vi "SA40144D.20210601 Devices + BG.vi"() -> ()   [LabVIEW 2020]
uses:
  <vilib>/Analysis/baseanly.llb/Mean (DBL).vi
  <userlib>/_OpenG.lib/file/file.llb/Build Path - Traditional__ogtk.vi
  <userlib>/LevyLab/LV to ITX/Data/Data.lvclass
  <userlib>/LevyLab/XY Utilities/xy_utilities.lvlib
  <vilib>/Analysis/NI_AALBase.lvlib
panel:
  in  "Tab Control":enum32{"Page 1", "Page 2", "Page 3"}(tab)
  out "G2T BG vs t":T1(graph)
  out "Temp vs t":T1(graph)
  out "G2T vs t 1D":T1(graph)
  out "G4T vs t 1D":T1(graph)
  out "G2T vs t 2D":T1(graph)
  out "G4T vs t  2D":T1(graph)
  out "Arrhenius":T1(graph)
  out "Lifespan vs Temp (hrs)":cluster{i32[], dbl[]}[](graph)
  out "Y3 2D I-":T1(graph)
  out "Y1 - BG I+":T1(graph)
  out "Y2 - 2D I+":T1(graph)
  out "Y4 - 1D I+":T1(graph)
  out "R3 - 2D I-":T1(graph)
  out "X3 - 2D I-":T1(graph)
  out "X2 - 2D I+":T1(graph)
  out "R1 - BG I+":T1(graph)
  out "X1 - BG I+":T1(graph)
  out "X4 - 1D I+":T1(graph)
  out "R2 - 2D I+":T1(graph)
  out "R4 - 1D I+":T1(graph)
  out "Y6 - 2D dV":T1(graph)
  out "Y8 - BG I-":T1(graph)
  out "Y5 - 1D I-":T1(graph)
  out "Y7 - 1D dV":T1(graph)
  out "R6 - 2D dV":T1(graph)
  out "R8 - BG I-":T1(graph)
  out "X5 - 1D I-":T1(graph)
  out "R5 - 1D I-":T1(graph)
  out "X6 - 2D dV":T1(graph)
  out "X7 - 1D dV":T1(graph)
  out "R7 - 1D dV":T1(graph)
  out "X8 - BG I-":T1(graph)
  in  "Toggle":bool
  in  "Temps to keep (Lifespan)":i32=26
  out "E_a":dbl[](array[numeric])
  in  "Temps to keep (Arrhenius fit)":i32=26
  in  "Source Voltage":dbl=0.1
  in  "Init Temp":i32=275
  in  "Temp Step":i32=5
  in  "Final Temp":i32=400
  in  "Data File":path=path "G:/My Drive/ansom/Data/PPMS 2/SA40144D.20210601/00 - Air Test/SA40144D.20210601.275K.dat"
  in  "Trimming":i32=400
  in  "Update":bool
  in  "OK":bool
  out "error out":errorcluster
  in  "error in (no error)":errorcluster
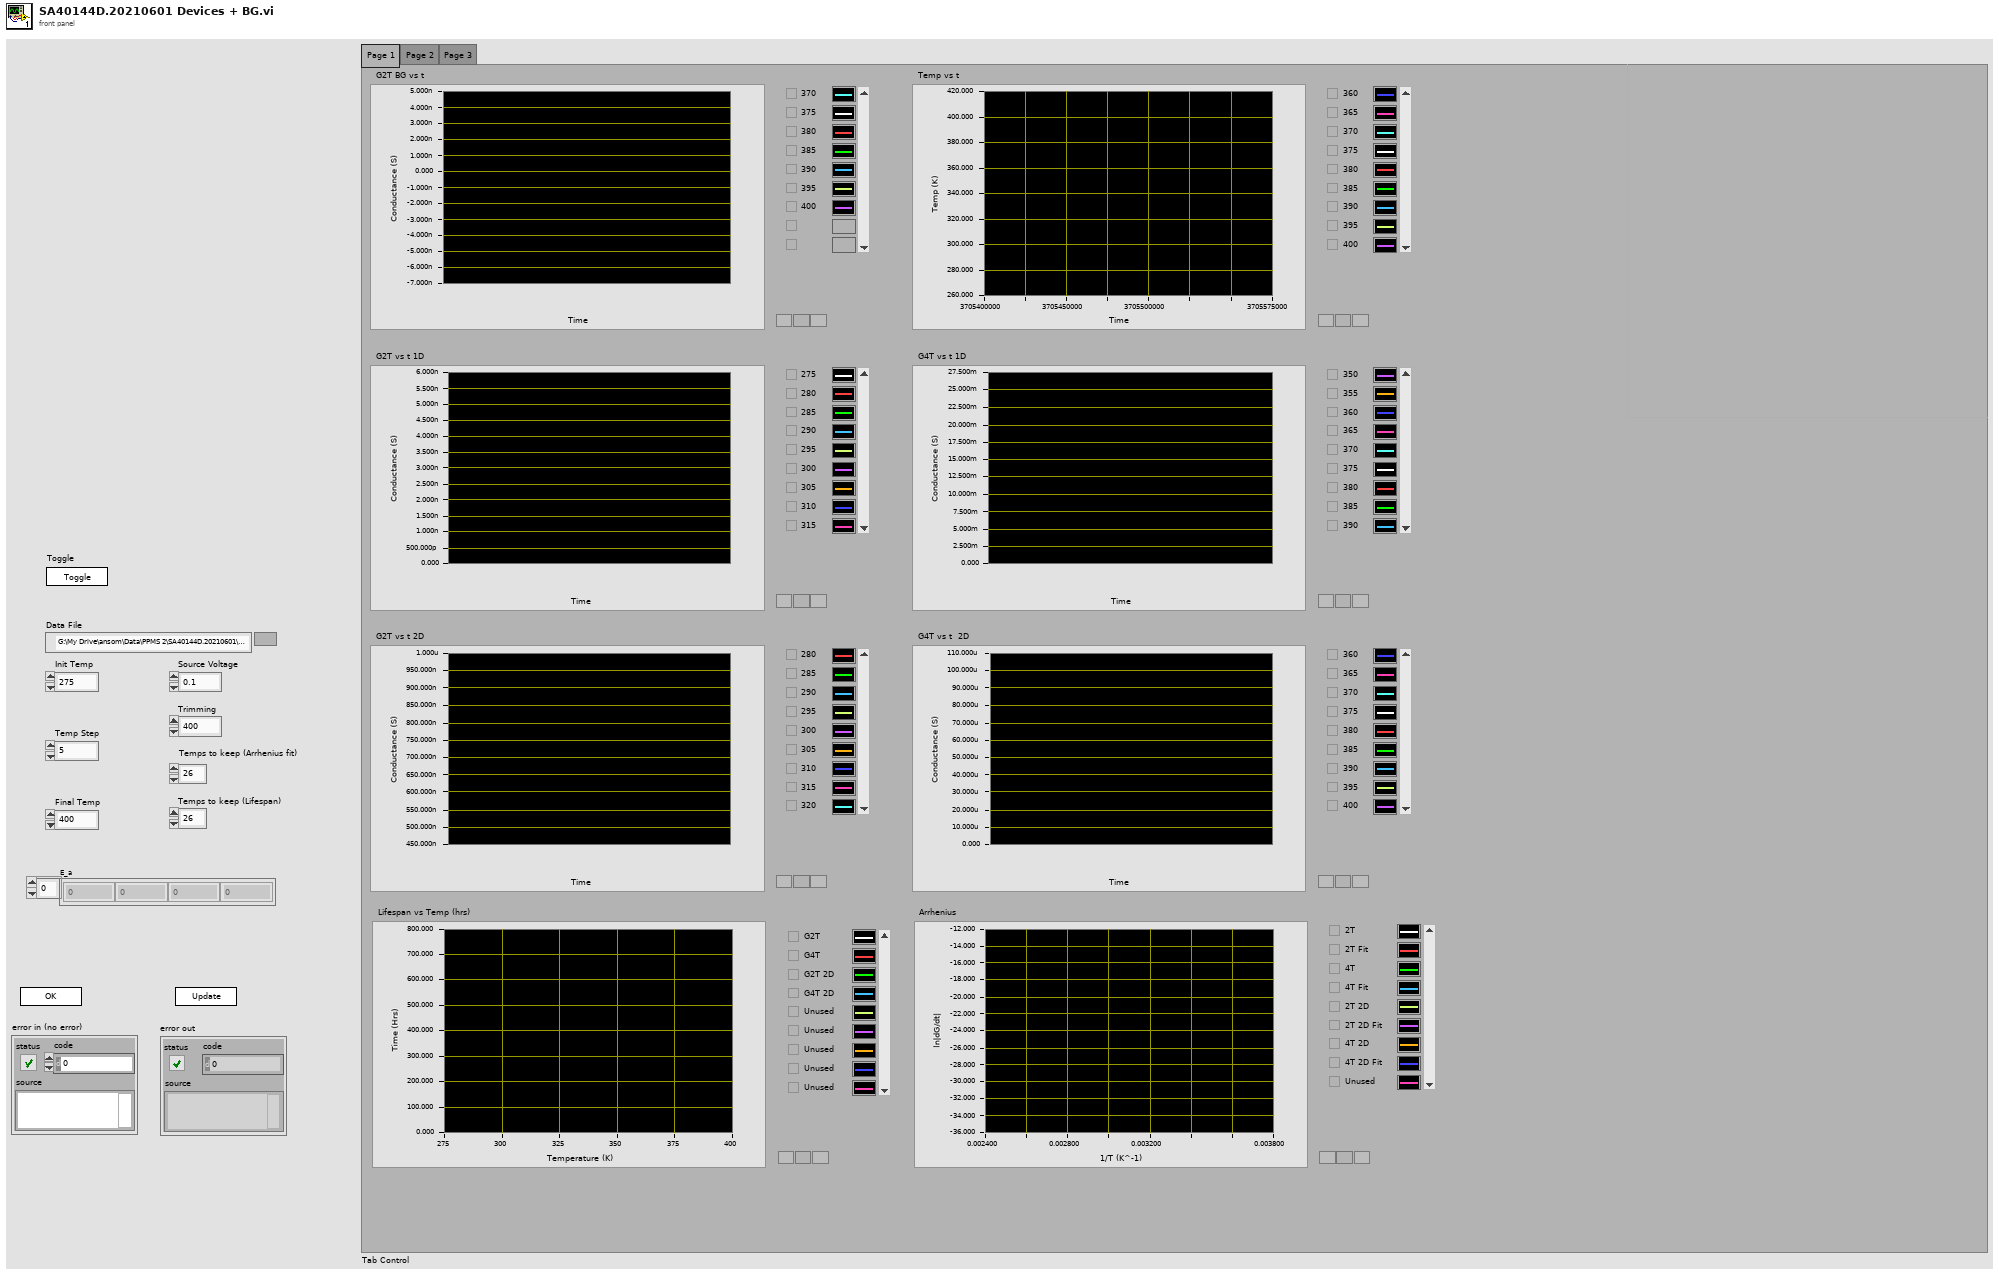
[diagram p1: front panel]
types:
  T1 = cluster{"Data":dbl[], "Best Exponential Fit":dbl[]}[]
  T2 = enum32{"Invalid", "Standard", "Closed", "Hidden", "Minimized", "Maximized"}
  T3 = enum32{"invalid app kind", "Development System", "Run Time System", "Student Edition", "Embedded LabVIEW", "Evaluation", "Custom"}
  T4 = cluster{"Core":cluster{"Current VI Reference":refnum<vi>, "Close Panel on Exit?":bool}, "G2T 1D":cluster{dbl[], dbl[]}[], "G4T 1D":cluster{dbl[], dbl[]}[], "G2T 2D":cluster{dbl[], dbl[]}[], "G4T 2D":cluster{dbl[], dbl[]}[], "Temp":cluster{dbl[], dbl[]}[], "G2T BG":cluster{dbl[], dbl[]}[], "Source Voltage":dbl, "Final Temp":i32, "Init Temp":i32, "Temp Step":i32, "Data File":path, "Trimming":i32}
  T5 = cluster{"Current VI Reference":refnum<vi>, "Close Panel on Exit?":bool}
  T6 = typedef "Data.lvclass/Dictionary--cluster.ctl" = cluster{"key":string, "value":variant}
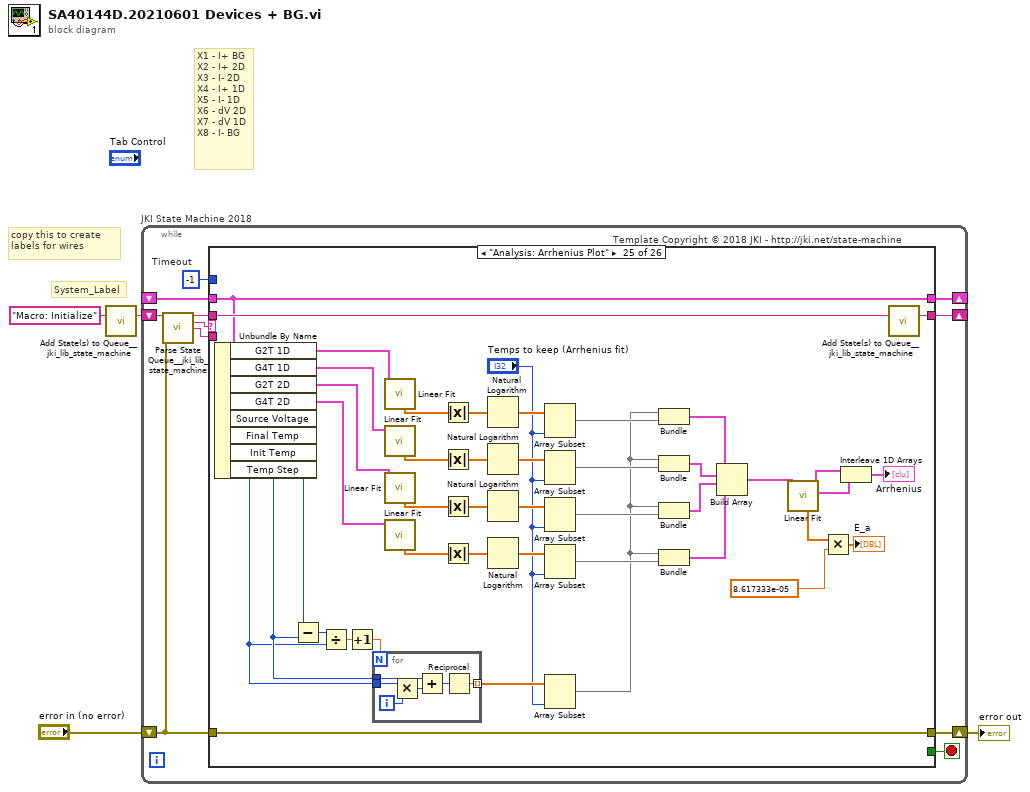
[diagram p0: block diagram]
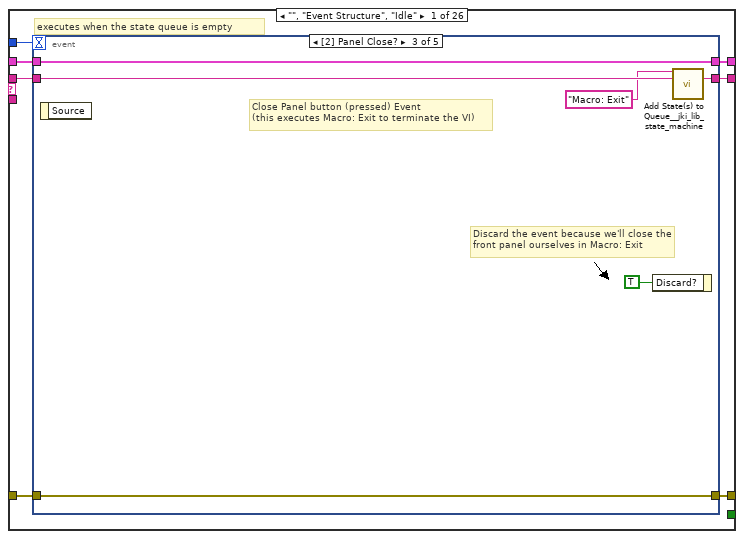
[diagram p2: hidden frame]
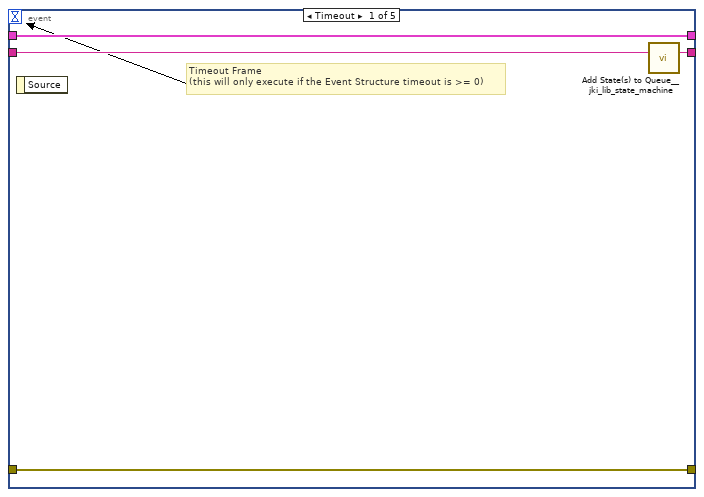
[diagram p3: hidden frame]
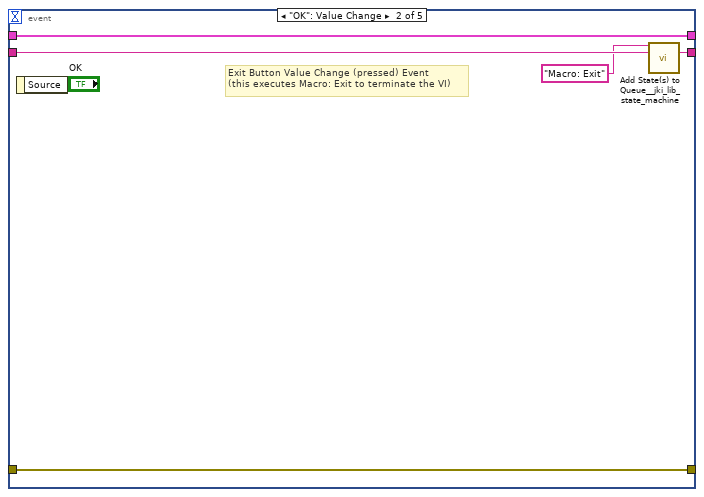
[diagram p4: hidden frame]
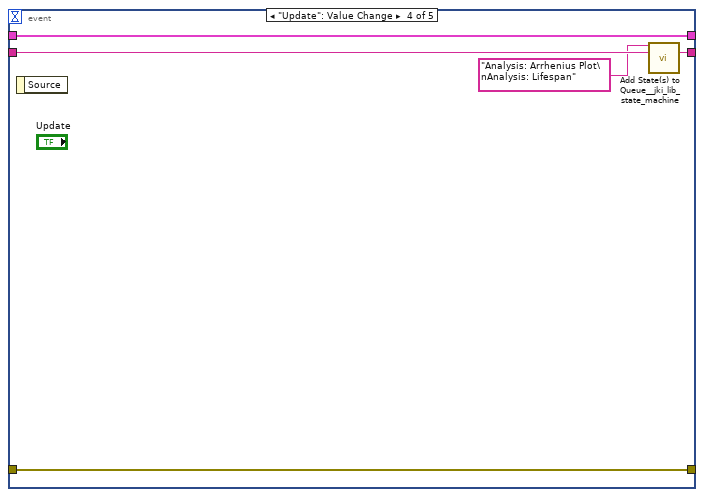
[diagram p5: hidden frame]
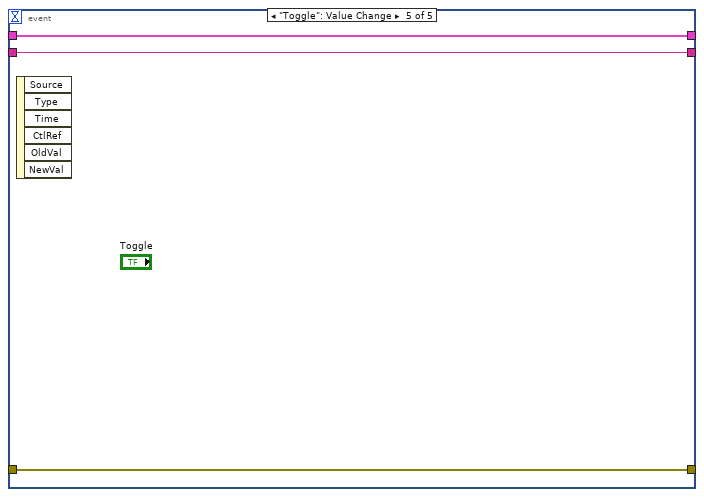
[diagram p6: hidden frame]
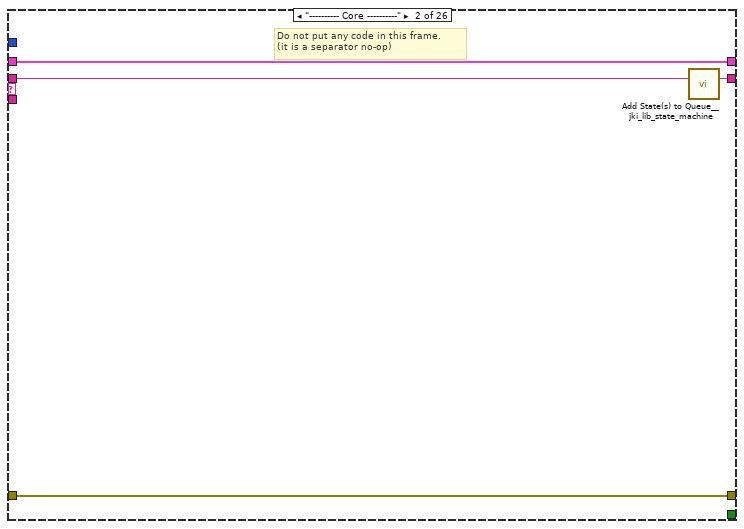
[diagram p7: hidden frame]
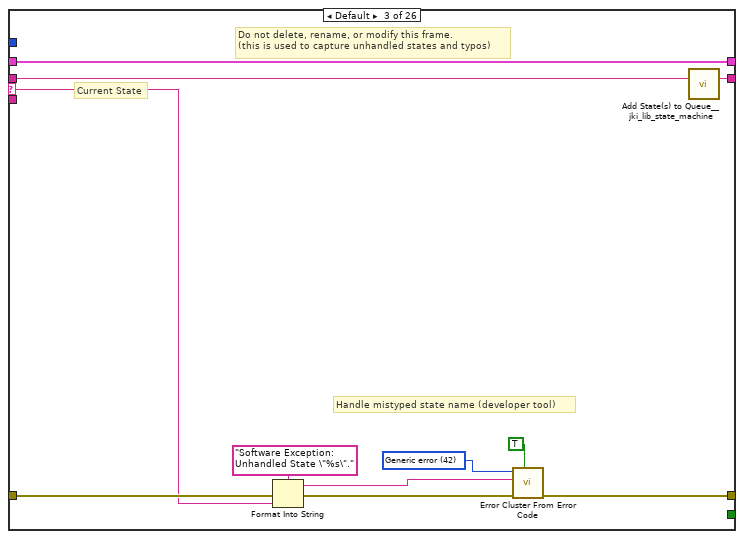
[diagram p8: hidden frame]
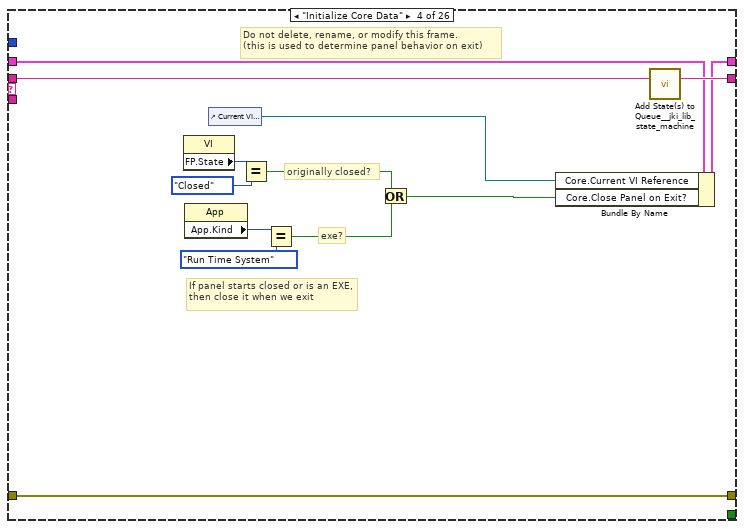
[diagram p9: hidden frame]
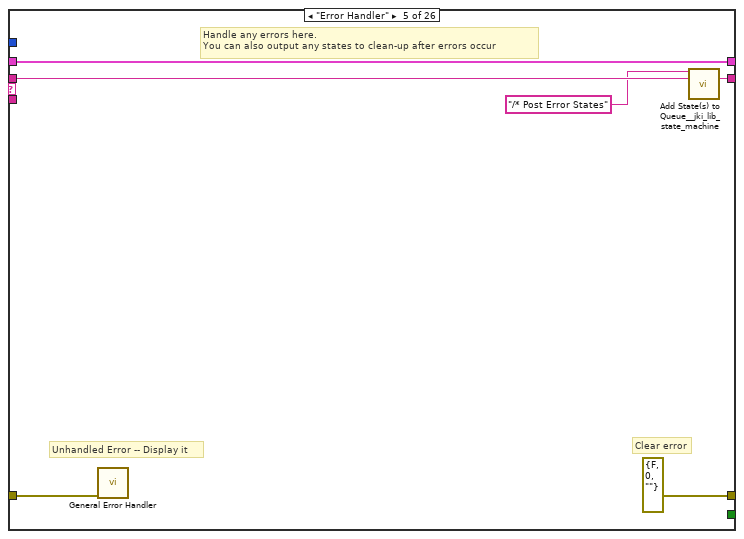
[diagram p10: hidden frame]
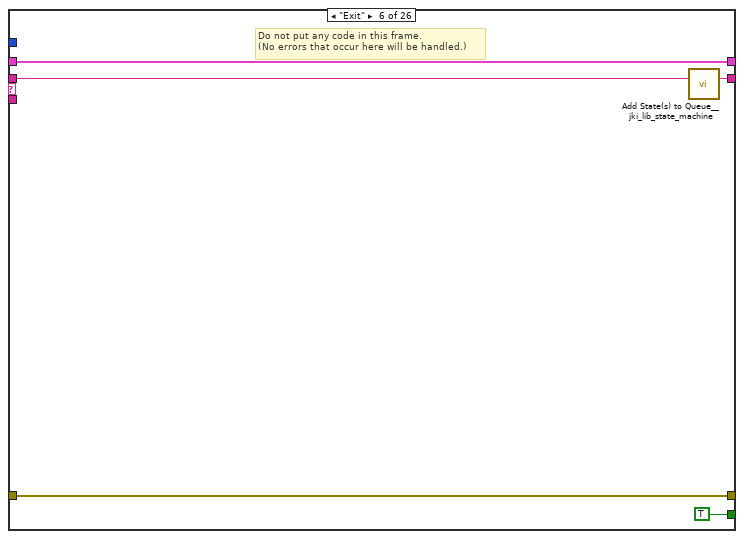
[diagram p11: hidden frame]
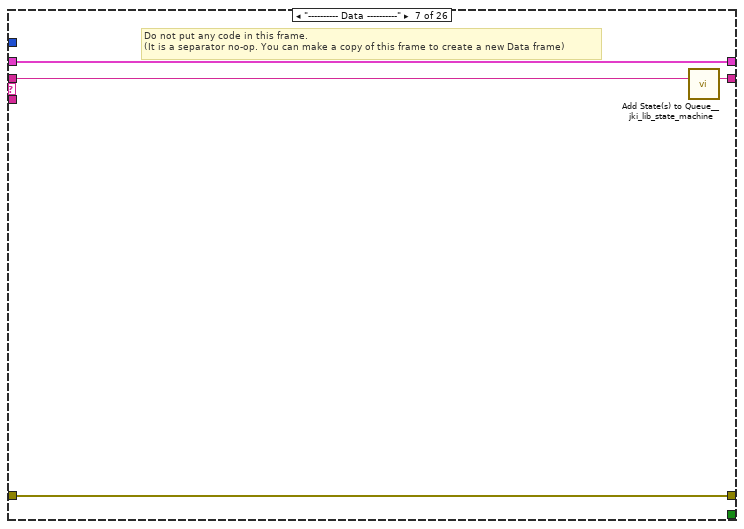
[diagram p12: hidden frame]
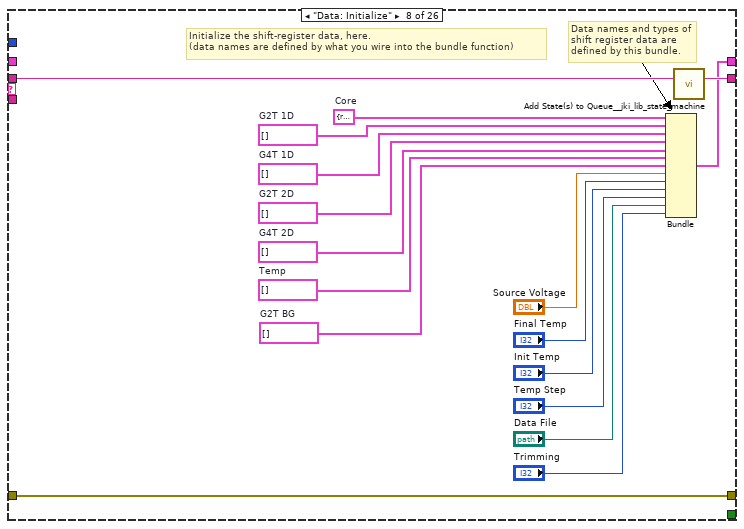
[diagram p13: hidden frame]
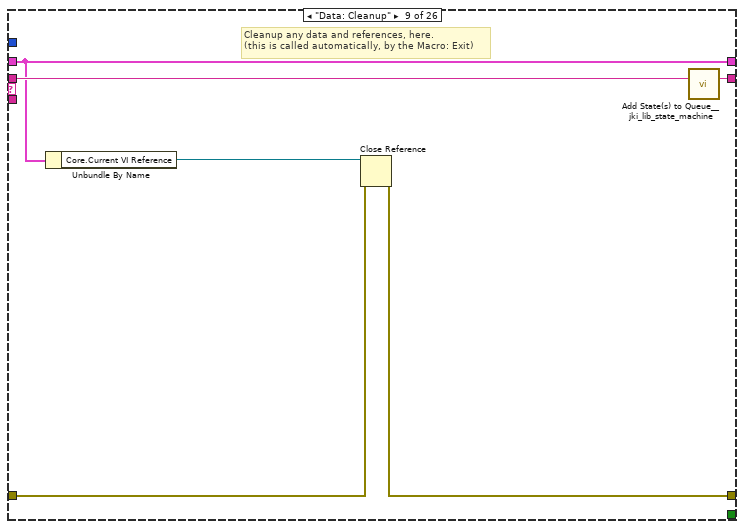
[diagram p14: hidden frame]
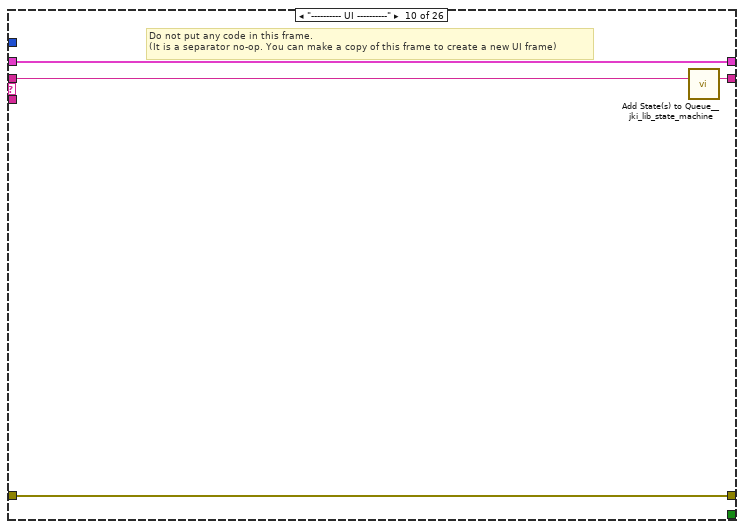
[diagram p15: hidden frame]
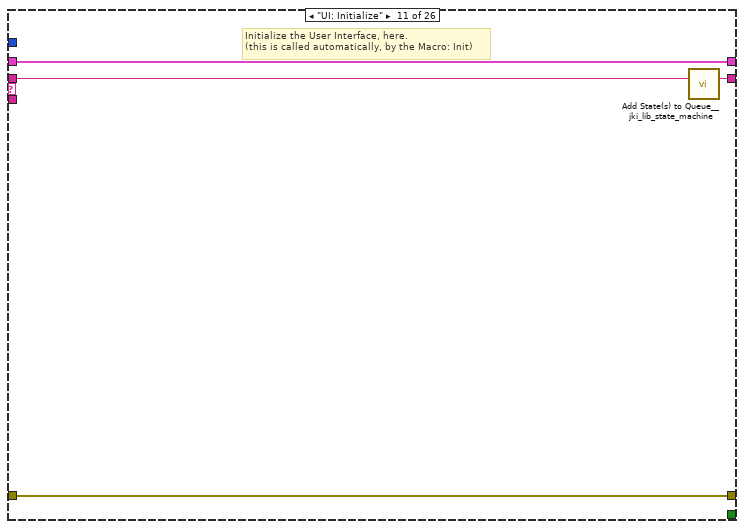
[diagram p16: hidden frame]
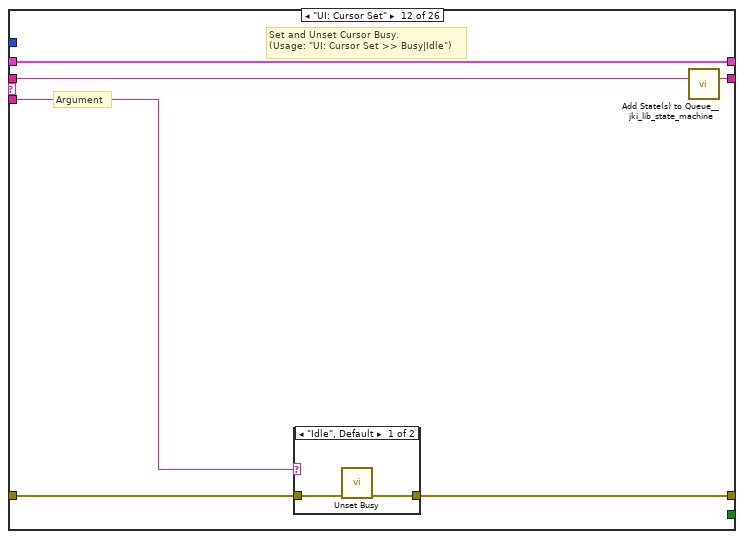
[diagram p17: hidden frame]
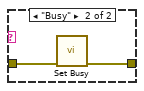
[diagram p18: hidden frame]
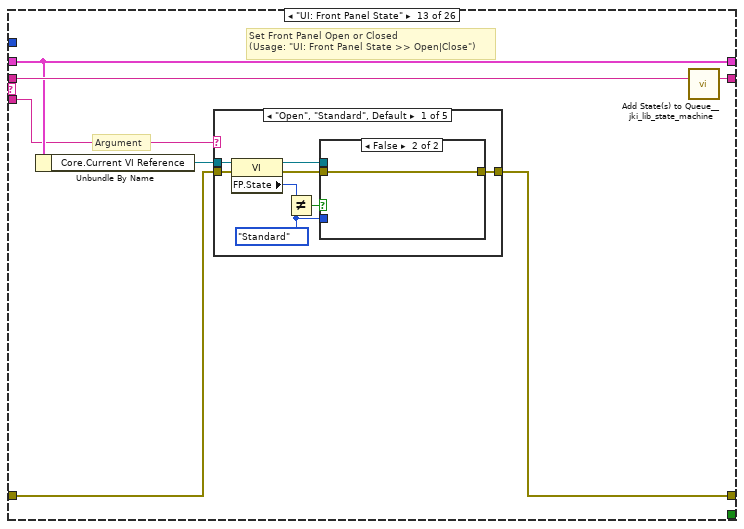
[diagram p19: hidden frame]
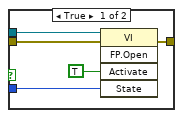
[diagram p20: hidden frame]
diagram:
  # "X1 - I+ BG\nX2 - I+ 2D\nX3 - I- 2D\nX4 - I+ 1D\nX5 - I- 1D\nX6 - dV 2D\nX7 - dV 1D\nX8 - I- BG"
  # "copy this to create labels for wires"
  # "System_Label"
  n1 = call <vilib>:"Add State(s) to Queue__jki_lib_state_machine.vi"("State(s) in (\"\")"="Macro: Initialize") -> ("States Out"=w4:string)  [unwired: 14 in]
  n2 = while "JKI State Machine 2018" {
    shift-right: [w8] -> _
    shift-left: _ -> [w7]
    shift-right: [w11] -> w1
    shift-left: "error in (no error)" -> [w5]
    shift-right: [w10] -> _
    shift-left: w4 -> [w12]
    stop <- w9 stop-if-true
    w6 = -1  # Timeout
    # "Template Copyright © 2018 JKI - http://jki.net/state-machine"
    n3 = call <vilib>:"Parse State Queue__jki_lib_state_machine.vi"("State Queue"=w12, "Error In (no error)"=w5) -> ("Remaining States"=w14:string, "Current State"=w15:string, "Arguments"=w13:string)  [unwired: 11 in]
    n4 = case shown="\"Analysis: Arrhenius Plot\"" w15 {
      selector: w15 -> [_ _ w50 _ _ _ _ _ _ _ _ _ _ _ _ _ _ _ _ _ _ _ _ _ _ _]
      tunnel: w14 -> [w22 w49 w54 w73 w79 w84 w88 w105 w111 w115 w119 w125 w136 w205 w210 w220 w224 w244 w314 w401 w485 w551 w598 w650 w694 w751]
      tunnel: w13 -> [_ _ _ _ _ _ _ _ _ _ _ w120 w130 _ _ _ _ _ _ _ _ _ _ _ _ _]
      tunnel: w7 -> [w20 w46 w52 w66 w76 w82 w85 _ w106 w112 w117 w123 w132 w202 w207 w217 w221 w241 w311 w398 w479 w536 w600 w647 w691 w731]
      tunnel: [w19 w47 w56 w70 errorcluster {"status"=FALSE, "code"=0, "source"=""} ("error out") w81 w86 w102 w107 w113 w116 w121 w133 w203 w208 w218 w222 w242 w312 w399 w481 w549 w612 w648 w692 w749] -> w11
      tunnel: w5 -> [w18 w47 w55 w70 w75 w81 w86 w102 w108 w113 w116 w122 w134 w203 w208 w218 w222 w242 w312 w399 w481 w549 w612 w648 w692 w749]
      tunnel: [w21 w48 w53 w72 w78 w83 w87 w104 w110 w114 w118 w124 w135 w204 w209 w219 w223 w243 w313 w400 w484 w550 w599 w649 w693 w750] -> w10
      tunnel: [_ _ _ _ _ TRUE _ _ _ _ _ _ _ _ _ _ _ _ _ _ _ _ _ _ _ _] -> w9
      tunnel: [w17 w46 w52 w71 w76 w82 w85 w103 w106 w112 w117 w123 w132 w202 w207 w217 w221 w241 w311 w398 w480 w537 w601 w647 w691 w731] -> w8
      tunnel: w6 -> [w16 _ _ _ _ _ _ _ _ _ _ _ _ _ _ _ _ _ _ _ _ _ _ _ _ _]
      frame "", "Event Structure", "Idle" {
        # "executes when the state queue is empty"
        n5 = event shown="[2] Panel Close?" {
          selector: _ -> [_ _ _ _ _]
          dyn-events: _ -> [_ _ _ _ _]
          timeout: w16 -> [_ _ _ _ _]
          tunnel: w22 -> [w26 w31 w37 w41 w44]
          tunnel: [w25 w30 w36 w40 w44] -> w21
          tunnel: w20 -> [w23 w28 w34 w42 w45]
          tunnel: [w24 w29 w35 w38 w43] -> w19
          tunnel: w18 -> [w24 w29 w35 w38 w43]
          tunnel: [w23 w28 w34 w42 w45] -> w17
          event Timeout {
            # "Timeout Frame\n(this will only execute if the Event Structure timeout is >= 0)"
            n6 = event-data() -> ()  [unwired: 1 in, 1 out]
            n7 = call <vilib>:"Add State(s) to Queue__jki_lib_state_machine.vi"("State(s) in (\"\")"=w26) -> ("States Out"=w25:string)  [unwired: 14 in]
          }
          event "OK": Value Change {
            # "Exit Button Value Change (pressed) Event\n(this executes Macro: Exit to terminate the VI)"
            n8 = event-data() -> ()  [unwired: 1 in, 1 out]
            n9 = call <vilib>:"Add State(s) to Queue__jki_lib_state_machine.vi"("State(s) in Front (\"\")"="Macro: Exit", "State(s) in (\"\")"=w31) -> ("States Out"=w30:string)  [unwired: 13 in]
          }
          event Panel Close? {
            # "Discard the event because we'll close the front panel ourselves in Macro: Exit"
            # "Close Panel button (pressed) Event\n(this executes Macro: Exit to terminate the VI)"
            n10 = event-data() -> ()  [unwired: 1 in, 1 out]
            n11 = event-data("Discard?"=TRUE) -> ()  [unwired: 1 in, 1 out]
            n12 = call <vilib>:"Add State(s) to Queue__jki_lib_state_machine.vi"("State(s) in Front (\"\")"="Macro: Exit", "State(s) in (\"\")"=w37) -> ("States Out"=w36:string)  [unwired: 13 in]
          }
          event "Update": Value Change {
            n13 = event-data() -> ()  [unwired: 1 in, 1 out]
            n14 = call <vilib>:"Add State(s) to Queue__jki_lib_state_machine.vi"("State(s) in Front (\"\")"="Analysis: Arrhenius Plot\nAnalysis: Lifespan" ("State(s) in Front (\"\")"), "State(s) in (\"\")"=w41) -> ("States Out"=w40:string)  [unwired: 13 in]
          }
          event "Toggle": Value Change {
            n15 = event-data() -> ()  [unwired: 1 in, 6 out]
          }
        }
      }
      frame "---------- Core ----------" {
        # "Do not put any code in this frame.\n(it is a separator no-op)"
        n16 = call <vilib>:"Add State(s) to Queue__jki_lib_state_machine.vi"("State(s) in (\"\")"=w49) -> ("States Out"=w48:string)  [unwired: 14 in]
      }
      frame Default {
        w59 = 42 items=["No error", "Argument error", "Memory is full", "Out of zone", "End of file", "File already open", "Generic file I/O error", "File not found", "File permission error", "Disk is full", "Duplicate path", "Too many files open", "System feature not enabled", "Resource file not found", "Cannot add resource", "Resource not found", "Image not found", "Image memory error", "Pen does not exist", "Config type invalid", "Config token not found", "Config parse error", "Config memory error", "Bad external code format", "Bad external code offset", "External code not present", "Null window", "Destroy window error", "Null menu", "Print aborted", "Bad print record", "Print driver error", "Windows error during printing", "Memory error during printing", "Print dialog error", "Generic print error", "Invalid device refnum", "Device not found", "Device parameter error", "Device unit error", "Cannot open device", "Device call aborted", "Generic error", "Cancelled by user", "Object ID too low", "Object ID too high", "Object not in heap", "Unknown heap", "Unknown object (invalid DefProc)", "Unknown object (DefProc not in table)", "Message out of range", "Invalid (null) method", "Unknown message", "Manager call not supported", "Bad address", "Network operation in progress", "Network operation timed out", "Connection is busy", "Network attribute not supported", "Network error", "Address in use", "System out of memory", "Connection aborted", "Connection refused", "Not connected", "Already connected", "Connection closed", "Initialization error (interapplication manager)", "Bad occurrence", "Wait on unbound occurrence handler", "Occurrence queue overflow", "Datalog type conflict", "Unused", "Unrecognized type (interapplication manager)", "Memory corrupt", "Failed to make temporary DLL", "Old CIN version", "Drag socket not found", "Failed to load drop-object", "Failed to register OLE object", "Failed to release OLE object", "Format specifier type mismatch", "Unknown format specifier", "Too few format specifiers", "Too many format specifiers", "Scan failed", "Newer CIN version", "Error converting to variant", "Runtime menu error", "Password tampered", "Variant attribute not found", "Incompatible variant data type", "Event data is not available", "Event Store is not present", "Occurrence is not found", "Event Queue is not created", "Event info is not available", "Refnum passed is NULL", "Error retrieving Class GUID", "Error retrieving CoClass GUID", "Error retrieving TypeLib GUID.", "Bad built application magic bytes.", "Specific driver is different from the specific driver associated with the Logical Name.", "There is no session opened to the class driver.", "Max Error", "MAX - Error with config objects", "MAX - Error loading configuration", "MAX - Group not supported"]
        # "Current State"
        # "Do not delete, rename, or modify this frame.\n(this is used to capture unhandled states and typos)"
        # "Handle mistyped state name (developer tool)"
        n17 = Format Into String(format string="Software Exception: Unhandled State \"%s\"." ("message"), error in=w55, w50) -> (resulting string=w58:string, error out=w57:errorcluster)  [unwired: 1 in]
        n18 = call <vilib>:"Error Cluster From Error Code.vi"("show call chain? (False)"=TRUE, "error in (no error)"=w57, "error message (\"\")"=w58, "error code (0)"=w59) -> ("error out"=w56:errorcluster)  [unwired: 5 in]
        n19 = call <vilib>:"Add State(s) to Queue__jki_lib_state_machine.vi"("State(s) in (\"\")"=w54) -> ("States Out"=w53:string)  [unwired: 14 in]
      }
      frame "Initialize Core Data" {
        # "Do not delete, rename, or modify this frame.\n(this is used to determine panel behavior on exit)"
        # "originally closed?"
        # "exe?"
        # "If panel starts closed or is an EXE, then close it when we exit"
        n20 = property class="VI"() -> ("FP.State"=w63:T2)  [unwired: 2 in, 2 out]
        n21 = property class="App"() -> ("App.Kind"=w69:T3)  [unwired: 2 in, 2 out]
        n22 = control-ref of="Current VI Reference"() -> (w64:refnum<vi>)
        n23 = Equal?(x=w63, y=T2."Closed" ("Front Panel Window:State")) -> (x = y?=w61:bool)
        n24 = Equal?(x=w69, y=T3."Run Time System" ("Application:Kind")) -> (x = y?=w67:bool)
        n25 = Or(x=w61, y=w67) -> (x .or. y?=w65:bool)
        n26 = Bundle By Name(cluster=w66, "Core.Current VI Reference"=w64, "Core.Close Panel on Exit?"=w65) -> (w71:T4)
        n27 = call <vilib>:"Add State(s) to Queue__jki_lib_state_machine.vi"("State(s) in (\"\")"=w73) -> ("States Out"=w72:string)  [unwired: 14 in]
      }
      frame "Error Handler" {
        # "Unhandled Error -- Display it"
        # "Handle any errors here.\nYou can also output any states to clean-up after errors occur"
        # "Clear error"
        n28 = call <vilib>:"General Error Handler.vi"("error in (no error)"=w75) -> ()  [unwired: 10 in, 5 out]
        n29 = call <vilib>:"Add State(s) to Queue__jki_lib_state_machine.vi"("State(s) in Front (\"\")"="/* Post Error States", "State(s) in (\"\")"=w79) -> ("States Out"=w78:string)  [unwired: 13 in]
      }
      frame "Exit" {
        # "Do not put any code in this frame.\n(No errors that occur here will be handled.)"
        n30 = call <vilib>:"Add State(s) to Queue__jki_lib_state_machine.vi"("State(s) in (\"\")"=w84) -> ("States Out"=w83:string)  [unwired: 14 in]
      }
      frame "---------- Data ----------" {
        # "Do not put any code in this frame.\n(It is a separator no-op. You can make a copy of this frame to create a new Data frame)"
        n31 = call <vilib>:"Add State(s) to Queue__jki_lib_state_machine.vi"("State(s) in (\"\")"=w88) -> ("States Out"=w87:string)  [unwired: 14 in]
      }
      frame "Data: Initialize" {
        w89 = cluster{dbl[], dbl[]}[] []  # G2T BG
        w90 = cluster{dbl[], dbl[]}[] []  # Temp
        w99 = cluster{dbl[], dbl[]}[] []  # G4T 2D
        w98 = cluster{dbl[], dbl[]}[] []  # G2T 2D
        w97 = cluster{dbl[], dbl[]}[] []  # G4T 1D
        w96 = cluster{dbl[], dbl[]}[] []  # G2T 1D
        w101 = T5 {"Current VI Reference"=refnum, "Close Panel on Exit?"=FALSE}  # Core
        # "Data names and types of shift register data are defined by this bundle."
        # "Initialize the shift-register data, here.\n(data names are defined by what you wire into the bundle function)"
        n32 = Bundle("Core"=w101, "G2T 1D"=w96, "G4T 1D"=w97, "G2T 2D"=w98, "G4T 2D"=w99, "Temp"=w90, "G2T BG"=w89, "Source Voltage"="Source Voltage", "Final Temp"="Final Temp", "Init Temp"="Init Temp", "Temp Step"="Temp Step", "Data File"="Data File", "Trimming"="Trimming") -> (w103:T4)  [unwired: 1 in]
        n33 = call <vilib>:"Add State(s) to Queue__jki_lib_state_machine.vi"("State(s) in (\"\")"=w105) -> ("States Out"=w104:string)  [unwired: 14 in]
      }
      frame "Data: Cleanup" {
        # "Cleanup any data and references, here.\n(this is called automatically, by the Macro: Exit)"
        n34 = Unbundle By Name(w106) -> ("Core.Current VI Reference"=w109:refnum<vi>)
        n35 = Close Reference(reference=w109, error in (no error)=w108) -> (error out=w107:errorcluster)
        n36 = call <vilib>:"Add State(s) to Queue__jki_lib_state_machine.vi"("State(s) in (\"\")"=w111) -> ("States Out"=w110:string)  [unwired: 14 in]
      }
      frame "---------- UI ----------" {
        # "Do not put any code in this frame.\n(It is a separator no-op. You can make a copy of this frame to create a new UI frame)"
        n37 = call <vilib>:"Add State(s) to Queue__jki_lib_state_machine.vi"("State(s) in (\"\")"=w115) -> ("States Out"=w114:string)  [unwired: 14 in]
      }
      frame "UI: Initialize" {
        # "Initialize the User Interface, here.\n(this is called automatically, by the Macro: Init)"
        n38 = call <vilib>:"Add State(s) to Queue__jki_lib_state_machine.vi"("State(s) in (\"\")"=w119) -> ("States Out"=w118:string)  [unwired: 14 in]
      }
      frame "UI: Cursor Set" {
        # "Argument"
        # "Set and Unset Cursor Busy.\n(Usage: \"UI: Cursor Set >> Busy|Idle\")"
        n39 = case shown="\"Idle\", Default" w120 {
          tunnel: w122 -> [w127 w129]
          tunnel: [w126 w128] -> w121
          frame "Idle", Default {
            n40 = call <vilib>:"Unset Busy.vi"("error in (no error)"=w127) -> ("error out"=w126:errorcluster)  [unwired: 10 in]
          }
          frame "Busy" {
            n41 = call <vilib>:"Set Busy.vi"("error in (no error)"=w129) -> ("error out"=w128:errorcluster)  [unwired: 9 in, 1 out]
          }
        }
        n42 = call <vilib>:"Add State(s) to Queue__jki_lib_state_machine.vi"("State(s) in (\"\")"=w125) -> ("States Out"=w124:string)  [unwired: 14 in]
      }
      frame "UI: Front Panel State" {
        # "Argument"
        # "Set Front Panel Open or Closed\n(Usage: \"UI: Front Panel State >> Open|Close\")"
        n43 = Unbundle By Name(w132) -> ("Core.Current VI Reference"=w131:refnum<vi>)
        n44 = case shown="\"Open\", \"Standard\", Default" w130 {
          tunnel: w134 -> [w142 w157 w168 w181 w194]
          tunnel: [w144 w158 w170 w183 w196] -> w133
          tunnel: w131 -> [w143 w155 w169 w182 w195]
          frame "Open", "Standard", Default {
            w137 = T2."Standard" ("State")
            n45 = property class="VI"(reference=w143, error in=w142) -> (reference out=w140:refnum<vi>, error out=w141:errorcluster, "FP.State"=w139:T2)
            n46 = Not Equal?(x=w139, y=w137) -> (x != y?=w138:bool)
            n47 = case shown="False" w138 {
              tunnel: [w148 w150] -> w144
              tunnel: w141 -> [w147 w150]
              tunnel: w140 -> [w146 _]
              tunnel: w137 -> [w145 _]
              frame True {
                n48 = invoke class="VI" method="FP.Open"(reference=w146, error in=w147, "Activate"=TRUE, "State"=w145) -> (error out=w148:errorcluster)  [unwired: 1 in, 4 out]
              }
              frame False {
              }
            }
          }
          frame "Close", "Closed" {
            n49 = property class="VI"(reference=w155, error in=w157) -> (reference out=w154:refnum<vi>, error out=w156:errorcluster, "FP.State"=w152:T2)
            n50 = Not Equal?(x=w152, y=T2."Closed" ("Front Panel Window:State")) -> (x != y?=w151:bool)
            n51 = case shown="True" w151 {
              tunnel: [w159 w162] -> w158
              tunnel: w156 -> [w159 w161]
              tunnel: w154 -> [_ w160]
              frame False {
              }
              frame True {
                n52 = invoke class="VI" method="FP.Close"(reference=w160, error in=w161) -> (error out=w162:errorcluster)  [unwired: 1 in, 2 out]
              }
            }
          }
          frame "Hidden", "Hide" {
            w163 = T2."Hidden" ("State")
            n53 = property class="VI"(reference=w169, error in=w168) -> (reference out=w166:refnum<vi>, error out=w167:errorcluster, "FP.State"=w165:T2)
            n54 = Not Equal?(x=w165, y=w163) -> (x != y?=w164:bool)
            n55 = case shown="True" w164 {
              tunnel: [w174 w175] -> w170
              tunnel: w167 -> [w173 w175]
              tunnel: w166 -> [w172 _]
              tunnel: w163 -> [w171 _]
              frame True {
                n56 = invoke class="VI" method="FP.Open"(reference=w172, error in=w173, "State"=w171) -> (error out=w174:errorcluster)  [unwired: 2 in, 4 out]
              }
              frame False {
              }
            }
          }
          frame "Minimize", "Minimized" {
            w176 = T2."Minimized" ("State")
            n57 = property class="VI"(reference=w182, error in=w181) -> (reference out=w179:refnum<vi>, error out=w180:errorcluster, "FP.State"=w178:T2)
            n58 = Not Equal?(x=w178, y=w176) -> (x != y?=w177:bool)
            n59 = case shown="True" w177 {
              tunnel: [w187 w188] -> w183
              tunnel: w180 -> [w186 w188]
              tunnel: w179 -> [w185 _]
              tunnel: w176 -> [w184 _]
              frame True {
                n60 = invoke class="VI" method="FP.Open"(reference=w185, error in=w186, "State"=w184) -> (error out=w187:errorcluster)  [unwired: 2 in, 4 out]
              }
              frame False {
              }
            }
          }
          frame "Maximize", "Maximized" {
            w189 = T2."Maximized" ("State")
            n61 = property class="VI"(reference=w195, error in=w194) -> (reference out=w192:refnum<vi>, error out=w193:errorcluster, "FP.State"=w191:T2)
            n62 = Not Equal?(x=w191, y=w189) -> (x != y?=w190:bool)
            n63 = case shown="True" w190 {
              tunnel: [w200 w201] -> w196
              tunnel: w193 -> [w199 w201]
              tunnel: w192 -> [w198 _]
              tunnel: w189 -> [w197 _]
              frame True {
                n64 = invoke class="VI" method="FP.Open"(reference=w198, error in=w199, "State"=w197) -> (error out=w200:errorcluster)  [unwired: 2 in, 4 out]
              }
              frame False {
              }
            }
          }
        }
        n65 = call <vilib>:"Add State(s) to Queue__jki_lib_state_machine.vi"("State(s) in (\"\")"=w136) -> ("States Out"=w135:string)  [unwired: 14 in]
      }
      frame "---------- Macro ----------" {
        # "Do not put any code in this frame.\n(It is a separator no-op. You can make a copy of this frame to create a new Macro frame)"
        n66 = call <vilib>:"Add State(s) to Queue__jki_lib_state_machine.vi"("State(s) in (\"\")"=w205) -> ("States Out"=w204:string)  [unwired: 14 in]
      }
      frame "Macro: Initialize" {
        # "Initialization Macro\n(This is called once, when the VI starts)"
        n67 = call <vilib>:"Add State(s) to Queue__jki_lib_state_machine.vi"("State(s) in Front (\"\")"="Data: Initialize\nInitialize Core Data\nUI: Initialize\nUI: Front Panel State >> Open\nAnalysis: Load 1D\nAnalysis: Load 2D\nAnalysis: Load BG\nAnalysis: X Data\nAnalysis: R Data\nAnalysis: R Data 2\nAnalysis: Plot G vs t\nAnalysis: Arrhenius Plot\nAnalysis: Lifespan", "State(s) in (\"\")"=w210) -> ("States Out"=w209:string)  [unwired: 13 in]
      }
      frame "Macro: Exit" {
        # "Exit Macro\n(This is called once, when the VI exits)"
        n68 = Unbundle By Name(w217) -> ("Core.Close Panel on Exit?"=w216:bool)
        n69 = Select(t="UI: Front Panel State >> Close", s=w216, f="") -> (s? t:f=w213:string)
        n70 = call <vilib>:"Add State(s) to Queue__jki_lib_state_machine.vi"("State(s) in (\"\")"=w213, "State(s) at Back (\"\")"="Data: Cleanup\nExit") -> ("States Out"=w211:string)  [unwired: 13 in]
        n71 = call <vilib>:"Add State(s) to Queue__jki_lib_state_machine.vi"("State(s) in Front (\"\")"=w211, "State(s) in (\"\")"=w220) -> ("States Out"=w219:string)  [unwired: 13 in]
      }
      frame "---------- Analysis ----------" {
        # "Template Separator\n(You can make a copy of, or modify, this frame)"
        n72 = call <vilib>:"Add State(s) to Queue__jki_lib_state_machine.vi"("State(s) in (\"\")"=w224) -> ("States Out"=w223:string)  [unwired: 14 in]
      }
      frame "Analysis: X Data" {
        # "Template Separator\n(You can make a copy of, or modify, this frame)"
        n73 = Unbundle By Name(w241) -> ("Final Temp"=w237:i32, "Init Temp"=w236:i32, "Temp Step"=w235:i32, "Data File"=w234:path, "Trimming"=w233:i32)
        n74 = Subtract(x=w237, y=w236) -> (x-y=w239:i32)
        n75 = Divide(x=w239, y=w235) -> (x/y=w240:dbl)
        n76 = Increment(x=w240) -> (x+1=w238:dbl)
        n77 = for {
          N: w238 -> [_]
          tunnel: w234 -> [w283]
          tunnel: w236 -> [w282]
          tunnel: w235 -> [w281]
          tunnel: w233 -> [w246]
          tunnel: [w257] -> w232 mode=indexing
          tunnel: [w256] -> w231 mode=indexing
          tunnel: [w255] -> w228 mode=indexing
          tunnel: [w254] -> w227 mode=indexing
          tunnel: [w249] -> w229 mode=indexing
          tunnel: [w248] -> w230 mode=indexing
          tunnel: [w247] -> w226 mode=indexing
          tunnel: [w245] -> w225 mode=indexing
          i -> [w285]
          n78 = Strip Path(path=w283) -> (stripped path=w290:path, name=w289:string)
          n79 = Multiply(x=w281, y=w285) -> (x*y=w286:i32)
          n80 = Add(x=w282, y=w286) -> (x+y=w291:i32)
          n81 = String Subset(string=w289, length (rest)=18) -> (substring=w287:string)  [unwired: 1 in]
          n82 = Format Into String(w291) -> (resulting string=w293:string)  [unwired: 3 in, 1 out]
          n83 = Concatenate Strings(w287, w293, "K.dat" ("string")) -> (w292:string)
          n84 = call-poly <userlib>:"Build Path__ogtk.vi"("name or relative path"=w292, "base path"=w290) -> ("appended path"=w294:path)
          n85 = call <userlib>:"Data Read.vi"("path"=w294) -> ("Data (Dictionary)"=w272:T6[])  [unwired: 7 in, 3 out]
          n86 = call "Read Dictionary.vi"("Numeric"=0, "Dictionary In"=w272) -> ("data"=w258:dbl[])
          n87 = call "Read Dictionary.vi"("Numeric"=3, "Dictionary In"=w272) -> ("data"=w273:dbl[])
          n88 = call "Read Dictionary.vi"("Numeric"=5, "Dictionary In"=w272) -> ("data"=w277:dbl[])
          n89 = call "Read Dictionary.vi"("Numeric"=7, "Dictionary In"=w272) -> ("data"=w279:dbl[])
          n90 = call "Read Dictionary.vi"("Numeric"=9, "Dictionary In"=w272) -> ("data"=w278:dbl[])
          n91 = Array Subset(array=w279, index=w246) -> (w265:dbl[])  [unwired: 1 in]
          n92 = Array Subset(array=w278, index=w246) -> (w266:dbl[])  [unwired: 1 in]
          n93 = Array Subset(array=w258, index=w246) -> ()  [unwired: 1 in, 1 out]
          n94 = Array Subset(array=w273, index=w246) -> (w263:dbl[])  [unwired: 1 in]
          n95 = Array Subset(array=w277, index=w246) -> (w264:dbl[])  [unwired: 1 in]
          n96 = Bundle("data"=w258, w263) -> (w257:cluster{"data":dbl[], dbl[]})  [unwired: 1 in]
          n97 = Bundle("data"=w258, w264) -> (w256:cluster{"data":dbl[], dbl[]})  [unwired: 1 in]
          n98 = Bundle("data"=w258, w265) -> (w255:cluster{"data":dbl[], dbl[]})  [unwired: 1 in]
          n99 = Bundle("data"=w258, w266) -> (w254:cluster{"data":dbl[], dbl[]})  [unwired: 1 in]
          n100 = call "Read Dictionary.vi"("Numeric"=4, "Dictionary In"=w272) -> ("data"=w271:dbl[])
          n101 = call "Read Dictionary.vi"("Numeric"=6, "Dictionary In"=w272) -> ("data"=w276:dbl[])
          n102 = call "Read Dictionary.vi"("Numeric"=8, "Dictionary In"=w272) -> ("data"=w274:dbl[])
          n103 = call "Read Dictionary.vi"("Numeric"=10, "Dictionary In"=w272) -> ("data"=w275:dbl[])
          n104 = Array Subset(array=w271, index=w246) -> (w262:dbl[])  [unwired: 1 in]
          n105 = Array Subset(array=w276, index=w246) -> (w261:dbl[])  [unwired: 1 in]
          n106 = Array Subset(array=w274, index=w246) -> (w260:dbl[])  [unwired: 1 in]
          n107 = Array Subset(array=w275, index=w246) -> (w259:dbl[])  [unwired: 1 in]
          n108 = Bundle("data"=w258, w259) -> (w245:cluster{"data":dbl[], dbl[]})  [unwired: 1 in]
          n109 = Bundle("data"=w258, w261) -> (w248:cluster{"data":dbl[], dbl[]})  [unwired: 1 in]
          n110 = Bundle("data"=w258, w260) -> (w247:cluster{"data":dbl[], dbl[]})  [unwired: 1 in]
          n111 = Bundle("data"=w258, w262) -> (w249:cluster{"data":dbl[], dbl[]})  [unwired: 1 in]
        }
        "X1 - BG I+" <- w232
        "X3 - 2D I-" <- w231
        "X4 - 1D I+" <- w230
        "X2 - 2D I+" <- w229
        "X5 - 1D I-" <- w228
        "X7 - 1D dV" <- w227
        "X8 - BG I-" <- w225
        "X6 - 2D dV" <- w226
        n112 = call <vilib>:"Add State(s) to Queue__jki_lib_state_machine.vi"("State(s) in (\"\")"=w244) -> ("States Out"=w243:string)  [unwired: 14 in]
      }
      frame "Analysis: R Data" {
        # "Template Separator\n(You can make a copy of, or modify, this frame)"
        n113 = Unbundle By Name(w311) -> ("Final Temp"=w307:i32, "Init Temp"=w306:i32, "Temp Step"=w305:i32, "Data File"=w304:path, "Trimming"=w303:i32)
        n114 = Subtract(x=w307, y=w306) -> (x-y=w309:i32)
        n115 = Divide(x=w309, y=w305) -> (x/y=w310:dbl)
        n116 = Increment(x=w310) -> (x+1=w308:dbl)
        n117 = for {
          N: w308 -> [_]
          tunnel: w304 -> [w370]
          tunnel: w306 -> [w369]
          tunnel: w305 -> [w368]
          tunnel: w303 -> [w345]
          tunnel: [w358] -> w302 mode=indexing
          tunnel: [w357] -> w301 mode=indexing
          tunnel: [w356] -> w300 mode=indexing
          tunnel: [w355] -> w299 mode=indexing
          tunnel: [w318] -> w298 mode=indexing
          tunnel: [w317] -> w297 mode=indexing
          tunnel: [w316] -> w296 mode=indexing
          tunnel: [w315] -> w295 mode=indexing
          i -> [w372]
          n118 = Strip Path(path=w370) -> (stripped path=w377:path, name=w376:string)
          n119 = Multiply(x=w368, y=w372) -> (x*y=w373:i32)
          n120 = Add(x=w369, y=w373) -> (x+y=w378:i32)
          n121 = String Subset(string=w376, length (rest)=18) -> (substring=w374:string)  [unwired: 1 in]
          n122 = Format Into String(w378) -> (resulting string=w380:string)  [unwired: 3 in, 1 out]
          n123 = Concatenate Strings(w374, w380, "K.dat" ("string")) -> (w379:string)
          n124 = call-poly <userlib>:"Build Path__ogtk.vi"("name or relative path"=w379, "base path"=w377) -> ("appended path"=w381:path)
          n125 = call <userlib>:"Data Read.vi"("path"=w381) -> ("Data (Dictionary)"=w350:T6[])  [unwired: 7 in, 3 out]
          n126 = call "Read Dictionary.vi"("Numeric"=0, "Dictionary In"=w350) -> ("data"=w324:dbl[])
          n127 = call "Read Dictionary.vi"("Numeric"=3, "Dictionary In"=w350) -> ("data"=w363:dbl[])
          n128 = call "Read Dictionary.vi"("Numeric"=5, "Dictionary In"=w350) -> ("data"=w364:dbl[])
          n129 = call "Read Dictionary.vi"("Numeric"=7, "Dictionary In"=w350) -> ("data"=w366:dbl[])
          n130 = call "Read Dictionary.vi"("Numeric"=9, "Dictionary In"=w350) -> ("data"=w365:dbl[])
          n131 = Array Subset(array=w366, index=w345) -> (w326:dbl[])  [unwired: 1 in]
          n132 = Array Subset(array=w365, index=w345) -> (w325:dbl[])  [unwired: 1 in]
          n133 = Array Subset(array=w324, index=w345) -> (w319:dbl[])  [unwired: 1 in]
          n134 = Array Subset(array=w363, index=w345) -> (w328:dbl[])  [unwired: 1 in]
          n135 = Array Subset(array=w364, index=w345) -> (w327:dbl[])  [unwired: 1 in]
          n136 = call "Read Dictionary.vi"("Numeric"=11, "Dictionary In"=w350) -> ("data"=w349:dbl[])
          n137 = call "Read Dictionary.vi"("Numeric"=13, "Dictionary In"=w350) -> ("data"=w348:dbl[])
          n138 = call "Read Dictionary.vi"("Numeric"=15, "Dictionary In"=w350) -> ("data"=w347:dbl[])
          n139 = call "Read Dictionary.vi"("Numeric"=17, "Dictionary In"=w350) -> ("data"=w346:dbl[])
          n140 = Array Subset(array=w349, index=w345) -> (w320:dbl[])  [unwired: 1 in]
          n141 = Array Subset(array=w348, index=w345) -> (w321:dbl[])  [unwired: 1 in]
          n142 = Array Subset(array=w347, index=w345) -> (w322:dbl[])  [unwired: 1 in]
          n143 = Array Subset(array=w346, index=w345) -> (w323:dbl[])  [unwired: 1 in]
          n144 = Bundle(w319, w320) -> (w318:cluster{dbl[], dbl[]})  [unwired: 1 in]
          n145 = Bundle(w319, w321) -> (w317:cluster{dbl[], dbl[]})  [unwired: 1 in]
          n146 = Bundle(w319, w322) -> (w316:cluster{dbl[], dbl[]})  [unwired: 1 in]
          n147 = Bundle(w319, w323) -> (w315:cluster{dbl[], dbl[]})  [unwired: 1 in]
          n148 = Square(x=w328) -> (x^2=w339:dbl[])
          n149 = Square(x=w320) -> (x^2=w340:dbl[])
          n150 = Square(x=w327) -> (x^2=w338:dbl[])
          n151 = Square(x=w321) -> (x^2=w337:dbl[])
          n152 = Square(x=w326) -> (x^2=w342:dbl[])
          n153 = Square(x=w322) -> (x^2=w341:dbl[])
          n154 = Square(x=w325) -> (x^2=w344:dbl[])
          n155 = Square(x=w323) -> (x^2=w343:dbl[])
          n156 = Add(x=w339, y=w340) -> (x+y=w334:dbl[])
          n157 = Add(x=w338, y=w337) -> (x+y=w333:dbl[])
          n158 = Add(x=w342, y=w341) -> (x+y=w335:dbl[])
          n159 = Add(x=w344, y=w343) -> (x+y=w336:dbl[])
          n160 = Square Root(x=w334) -> (sqrt(x)=w332:dbl[])
          n161 = Square Root(x=w333) -> (sqrt(x)=w331:dbl[])
          n162 = Square Root(x=w335) -> (sqrt(x)=w330:dbl[])
          n163 = Square Root(x=w336) -> (sqrt(x)=w329:dbl[])
          n164 = Bundle(w319, w332) -> (w358:cluster{dbl[], dbl[]})  [unwired: 1 in]
          n165 = Bundle(w319, w331) -> (w357:cluster{dbl[], dbl[]})  [unwired: 1 in]
          n166 = Bundle(w319, w330) -> (w356:cluster{dbl[], dbl[]})  [unwired: 1 in]
          n167 = Bundle(w319, w329) -> (w355:cluster{dbl[], dbl[]})  [unwired: 1 in]
        }
        "R1 - BG I+" <- w302
        "R3 - 2D I-" <- w301
        "R5 - 1D I-" <- w300
        "R7 - 1D dV" <- w299
        "Y1 - BG I+" <- w298
        "Y7 - 1D dV" <- w295
        "Y5 - 1D I-" <- w296
        "Y3 2D I-" <- w297
        n168 = call <vilib>:"Add State(s) to Queue__jki_lib_state_machine.vi"("State(s) in (\"\")"=w314) -> ("States Out"=w313:string)  [unwired: 14 in]
      }
      frame "Analysis: R Data 2" {
        # "Template Separator\n(You can make a copy of, or modify, this frame)"
        n169 = Unbundle By Name(w398) -> ("Final Temp"=w394:i32, "Init Temp"=w393:i32, "Temp Step"=w392:i32, "Data File"=w391:path, "Trimming"=w390:i32)
        n170 = Subtract(x=w394, y=w393) -> (x-y=w396:i32)
        n171 = Divide(x=w396, y=w392) -> (x/y=w397:dbl)
        n172 = Increment(x=w397) -> (x+1=w395:dbl)
        n173 = for {
          N: w395 -> [_]
          tunnel: w391 -> [w457]
          tunnel: w393 -> [w456]
          tunnel: w392 -> [w455]
          tunnel: w390 -> [w432]
          tunnel: [w445] -> w389 mode=indexing
          tunnel: [w444] -> w388 mode=indexing
          tunnel: [w443] -> w387 mode=indexing
          tunnel: [w442] -> w386 mode=indexing
          tunnel: [w405] -> w385 mode=indexing
          tunnel: [w404] -> w384 mode=indexing
          tunnel: [w403] -> w383 mode=indexing
          tunnel: [w402] -> w382 mode=indexing
          i -> [w459]
          n174 = Strip Path(path=w457) -> (stripped path=w464:path, name=w463:string)
          n175 = Multiply(x=w455, y=w459) -> (x*y=w460:i32)
          n176 = Add(x=w456, y=w460) -> (x+y=w465:i32)
          n177 = String Subset(string=w463, length (rest)=18) -> (substring=w461:string)  [unwired: 1 in]
          n178 = Format Into String(w465) -> (resulting string=w467:string)  [unwired: 3 in, 1 out]
          n179 = Concatenate Strings(w461, w467, "K.dat" ("string")) -> (w466:string)
          n180 = call-poly <userlib>:"Build Path__ogtk.vi"("name or relative path"=w466, "base path"=w464) -> ("appended path"=w468:path)
          n181 = call <userlib>:"Data Read.vi"("path"=w468) -> ("Data (Dictionary)"=w437:T6[])  [unwired: 7 in, 3 out]
          n182 = call "Read Dictionary.vi"("Numeric"=0, "Dictionary In"=w437) -> ("data"=w413:dbl[])
          n183 = call "Read Dictionary.vi"("Numeric"=4, "Dictionary In"=w437) -> ("data"=w450:dbl[])
          n184 = call "Read Dictionary.vi"("Numeric"=6, "Dictionary In"=w437) -> ("data"=w451:dbl[])
          n185 = call "Read Dictionary.vi"("Numeric"=8, "Dictionary In"=w437) -> ("data"=w453:dbl[])
          n186 = call "Read Dictionary.vi"("Numeric"=10, "Dictionary In"=w437) -> ("data"=w452:dbl[])
          n187 = Array Subset(array=w453, index=w432) -> (w412:dbl[])  [unwired: 1 in]
          n188 = Array Subset(array=w452, index=w432) -> (w411:dbl[])  [unwired: 1 in]
          n189 = Array Subset(array=w413, index=w432) -> (w406:dbl[])  [unwired: 1 in]
          n190 = Array Subset(array=w450, index=w432) -> (w415:dbl[])  [unwired: 1 in]
          n191 = Array Subset(array=w451, index=w432) -> (w414:dbl[])  [unwired: 1 in]
          n192 = call "Read Dictionary.vi"("Numeric"=12, "Dictionary In"=w437) -> ("data"=w436:dbl[])
          n193 = call "Read Dictionary.vi"("Numeric"=14, "Dictionary In"=w437) -> ("data"=w435:dbl[])
          n194 = call "Read Dictionary.vi"("Numeric"=16, "Dictionary In"=w437) -> ("data"=w434:dbl[])
          n195 = call "Read Dictionary.vi"("Numeric"=18, "Dictionary In"=w437) -> ("data"=w433:dbl[])
          n196 = Array Subset(array=w436, index=w432) -> (w410:dbl[])  [unwired: 1 in]
          n197 = Array Subset(array=w435, index=w432) -> (w409:dbl[])  [unwired: 1 in]
          n198 = Array Subset(array=w434, index=w432) -> (w408:dbl[])  [unwired: 1 in]
          n199 = Array Subset(array=w433, index=w432) -> (w407:dbl[])  [unwired: 1 in]
          n200 = Bundle(w406, w409) -> (w404:cluster{dbl[], dbl[]})  [unwired: 1 in]
          n201 = Bundle(w406, w408) -> (w403:cluster{dbl[], dbl[]})  [unwired: 1 in]
          n202 = Bundle(w406, w407) -> (w402:cluster{dbl[], dbl[]})  [unwired: 1 in]
          n203 = Bundle(w406, w410) -> (w405:cluster{dbl[], dbl[]})  [unwired: 1 in]
          n204 = Square(x=w415) -> (x^2=w426:dbl[])
          n205 = Square(x=w410) -> (x^2=w427:dbl[])
          n206 = Square(x=w414) -> (x^2=w425:dbl[])
          n207 = Square(x=w409) -> (x^2=w424:dbl[])
          n208 = Square(x=w412) -> (x^2=w429:dbl[])
          n209 = Square(x=w408) -> (x^2=w428:dbl[])
          n210 = Square(x=w411) -> (x^2=w431:dbl[])
          n211 = Square(x=w407) -> (x^2=w430:dbl[])
          n212 = Add(x=w426, y=w427) -> (x+y=w421:dbl[])
          n213 = Add(x=w425, y=w424) -> (x+y=w420:dbl[])
          n214 = Add(x=w429, y=w428) -> (x+y=w422:dbl[])
          n215 = Add(x=w431, y=w430) -> (x+y=w423:dbl[])
          n216 = Square Root(x=w421) -> (sqrt(x)=w419:dbl[])
          n217 = Square Root(x=w420) -> (sqrt(x)=w418:dbl[])
          n218 = Square Root(x=w422) -> (sqrt(x)=w417:dbl[])
          n219 = Square Root(x=w423) -> (sqrt(x)=w416:dbl[])
          n220 = Bundle(w406, w419) -> (w445:cluster{dbl[], dbl[]})  [unwired: 1 in]
          n221 = Bundle(w406, w418) -> (w444:cluster{dbl[], dbl[]})  [unwired: 1 in]
          n222 = Bundle(w406, w417) -> (w443:cluster{dbl[], dbl[]})  [unwired: 1 in]
          n223 = Bundle(w406, w416) -> (w442:cluster{dbl[], dbl[]})  [unwired: 1 in]
        }
        "R2 - 2D I+" <- w389
        "R4 - 1D I+" <- w388
        "R8 - BG I-" <- w386
        "R6 - 2D dV" <- w387
        "Y2 - 2D I+" <- w385
        "Y4 - 1D I+" <- w384
        "Y6 - 2D dV" <- w383
        "Y8 - BG I-" <- w382
        n224 = call <vilib>:"Add State(s) to Queue__jki_lib_state_machine.vi"("State(s) in (\"\")"=w401) -> ("States Out"=w400:string)  [unwired: 14 in]
      }
      frame "Analysis: Load 1D" {
        n225 = Unbundle By Name(w479) -> ("Source Voltage"=w478:dbl, "Final Temp"=w475:i32, "Init Temp"=w472:i32, "Temp Step"=w471:i32, "Data File"=w473:path, "Trimming"=w470:i32)
        n226 = Subtract(x=w475, y=w472) -> (x-y=w482:i32)
        n227 = Divide(x=w482, y=w471) -> (x/y=w483:dbl)
        n228 = Increment(x=w483) -> (x+1=w474:dbl)
        n229 = for {
          N: w474 -> [_]
          tunnel: w478 -> [w510]
          tunnel: [w524] -> w477 mode=indexing
          tunnel: [w523] -> w476 mode=indexing
          tunnel: w473 -> [w522]
          tunnel: w472 -> [w521]
          tunnel: w471 -> [w520]
          tunnel: w470 -> [w519]
          tunnel: [w516] -> w469 mode=indexing
          i -> [w526]
          w505 = -10 ("right rank")
          w504 = 10 ("left rank")
          n230 = Multiply(x=w520, y=w526) -> (x*y=w527:i32)
          n231 = Strip Path(path=w522) -> (stripped path=w531:path, name=w530:string)
          n232 = Add(x=w521, y=w527) -> (x+y=w532:i32)
          n233 = String Subset(string=w530, length (rest)=18) -> (substring=w528:string)  [unwired: 1 in]
          n234 = Format Into String(w532) -> (resulting string=w534:string)  [unwired: 3 in, 1 out]
          n235 = Concatenate Strings(w528, w534, "K.dat" ("string")) -> (w533:string)
          n236 = call-poly <userlib>:"Build Path__ogtk.vi"("name or relative path"=w533, "base path"=w531) -> ("appended path"=w535:path)
          n237 = call <userlib>:"Data Read.vi"("path"=w535) -> ("Data (Dictionary)"=w486:T6[])  [unwired: 7 in, 3 out]
          n238 = call "Read Dictionary.vi"("Numeric"=7 ("index"), "Dictionary In"=w486) -> ("data"=w496:dbl[])
          n239 = call "Read Dictionary.vi"("Numeric"=15 ("index"), "Dictionary In"=w486) -> ("data"=w495:dbl[])
          n240 = call "Read Dictionary.vi"("Numeric"=9, "Dictionary In"=w486) -> ("data"=w489:dbl[])
          n241 = call "Read Dictionary.vi"("Numeric"=17, "Dictionary In"=w486) -> ("data"=w488:dbl[])
          n242 = call "Read Dictionary.vi"("Numeric"=1, "Dictionary In"=w486) -> ("data"=w512:dbl[])
          n243 = call "Read Dictionary.vi"("Numeric"=0, "Dictionary In"=w486) -> ("data"=w513:dbl[])
          n244 = Square(x=w488) -> (x^2=w492:dbl[])
          n245 = Square(x=w489) -> (x^2=w491:dbl[])
          n246 = Square(x=w496) -> (x^2=w499:dbl[])
          n247 = Square(x=w495) -> (x^2=w500:dbl[])
          n248 = Add(x=w491, y=w492) -> (x+y=w490:dbl[])
          n249 = Add(x=w499, y=w500) -> (x+y=w498:dbl[])
          n250 = Square Root(x=w490) -> (sqrt(x)=w487:dbl[])
          n251 = Square Root(x=w498) -> (sqrt(x)=w497:dbl[])
          n252 = Array Subset(array=w512) -> (w517:dbl[])  [unwired: 2 in]
          n253 = Array Subset(array=w513, index=w519) -> (w518:dbl[])  [unwired: 1 in]
          n254 = Array Subset(array=w497, index=w519) -> (w509:dbl[])  [unwired: 1 in]
          n255 = Array Subset(array=w487, index=w519) -> (w508:dbl[])  [unwired: 1 in]
          n256 = Divide(x=w509, y=w510) -> (x/y=w503:dbl[])
          n257 = Divide(x=w509, y=w508) -> (x/y=w502:dbl[])
          n258 = call <vilib>:"Median Filter.vi"("right rank"=w505, "left rank"=w504, "X"=w503) -> ("Filtered X"=w507:dbl[])  [unwired: 7 in, 1 out]
          n259 = call <vilib>:"Median Filter.vi"("right rank"=w505, "left rank"=w504, "X"=w502) -> ("Filtered X"=w506:dbl[])  [unwired: 7 in, 1 out]
          n260 = Bundle(w518, "Filtered X"=w507) -> (w524:cluster{dbl[], "Filtered X":dbl[]})  [unwired: 1 in]
          n261 = Bundle(w518, w517) -> (w516:cluster{dbl[], dbl[]})  [unwired: 1 in]
          n262 = Bundle(w518, "Filtered X"=w506) -> (w523:cluster{dbl[], "Filtered X":dbl[]})  [unwired: 1 in]
        }
        n263 = call <vilib>:"Add State(s) to Queue__jki_lib_state_machine.vi"("State(s) in (\"\")"=w485) -> ("States Out"=w484:string)  [unwired: 14 in]
        n264 = Bundle By Name(cluster=w479, "G2T 1D"=w477, "G4T 1D"=w476, "Temp"=w469) -> (w480:T4)
      }
      frame "Analysis: Load 2D" {
        n265 = Unbundle By Name(w536) -> ("Source Voltage"=w546:dbl, "Final Temp"=w543:i32, "Init Temp"=w540:i32, "Temp Step"=w539:i32, "Data File"=w541:path, "Trimming"=w538:i32)
        n266 = Subtract(x=w543, y=w540) -> (x-y=w547:i32)
        n267 = Divide(x=w547, y=w539) -> (x/y=w548:dbl)
        n268 = Increment(x=w548) -> (x+1=w542:dbl)
        n269 = for {
          N: w542 -> [_]
          tunnel: w546 -> [w575]
          tunnel: [w586] -> w545 mode=indexing
          tunnel: [w585] -> w544 mode=indexing
          tunnel: w541 -> [w584]
          tunnel: w540 -> [w583]
          tunnel: w539 -> [w582]
          tunnel: w538 -> [w581]
          i -> [w588]
          w568 = -10 ("right rank")
          w569 = 10 ("left rank")
          n270 = Strip Path(path=w584) -> (stripped path=w593:path, name=w592:string)
          n271 = Multiply(x=w582, y=w588) -> (x*y=w589:i32)
          n272 = Add(x=w583, y=w589) -> (x+y=w594:i32)
          n273 = String Subset(string=w592, length (rest)=18) -> (substring=w590:string)  [unwired: 1 in]
          n274 = Format Into String(w594) -> (resulting string=w596:string)  [unwired: 3 in, 1 out]
          n275 = Concatenate Strings(w590, w596, "K.dat" ("string")) -> (w595:string)
          n276 = call-poly <userlib>:"Build Path__ogtk.vi"("name or relative path"=w595, "base path"=w593) -> ("appended path"=w597:path)
          n277 = call <userlib>:"Data Read.vi"("path"=w597) -> ("Data (Dictionary)"=w554:T6[])  [unwired: 7 in, 3 out]
          n278 = call "Read Dictionary.vi"("Numeric"=0, "Dictionary In"=w554) -> ("data"=w555:dbl[])
          n279 = call "Read Dictionary.vi"("Numeric"=6, "Dictionary In"=w554) -> ("data"=w558:dbl[])
          n280 = call "Read Dictionary.vi"("Numeric"=14 ("index"), "Dictionary In"=w554) -> ("data"=w557:dbl[])
          n281 = call "Read Dictionary.vi"("Numeric"=8, "Dictionary In"=w554) -> ("data"=w563:dbl[])
          n282 = call "Read Dictionary.vi"("Numeric"=16, "Dictionary In"=w554) -> ("data"=w564:dbl[])
          n283 = Square(x=w558) -> (x^2=w560:dbl[])
          n284 = Square(x=w557) -> (x^2=w561:dbl[])
          n285 = Square(x=w563) -> (x^2=w566:dbl[])
          n286 = Square(x=w564) -> (x^2=w567:dbl[])
          n287 = Add(x=w560, y=w561) -> (x+y=w559:dbl[])
          n288 = Add(x=w566, y=w567) -> (x+y=w565:dbl[])
          n289 = Square Root(x=w559) -> (sqrt(x)=w556:dbl[])
          n290 = Square Root(x=w565) -> (sqrt(x)=w562:dbl[])
          n291 = Array Subset(array=w555, index=w581) -> (w580:dbl[])  [unwired: 1 in]
          n292 = Array Subset(array=w556, index=w581) -> (w576:dbl[])  [unwired: 1 in]
          n293 = Array Subset(array=w562, index=w581) -> (w574:dbl[])  [unwired: 1 in]
          n294 = Divide(x=w576, y=w575) -> (x/y=w573:dbl[])
          n295 = Divide(x=w576, y=w574) -> (x/y=w571:dbl[])
          n296 = call <vilib>:"Median Filter.vi"("right rank"=w568, "left rank"=w569, "X"=w573) -> ("Filtered X"=w572:dbl[])  [unwired: 7 in, 1 out]
          n297 = call <vilib>:"Median Filter.vi"("right rank"=w568, "left rank"=w569, "X"=w571) -> ("Filtered X"=w570:dbl[])  [unwired: 7 in, 1 out]
          n298 = Bundle(w580, "Filtered X"=w572) -> (w586:cluster{dbl[], "Filtered X":dbl[]})  [unwired: 1 in]
          n299 = Bundle(w580, "Filtered X"=w570) -> (w585:cluster{dbl[], "Filtered X":dbl[]})  [unwired: 1 in]
        }
        n300 = call <vilib>:"Add State(s) to Queue__jki_lib_state_machine.vi"("State(s) in (\"\")"=w551) -> ("States Out"=w550:string)  [unwired: 14 in]
        n301 = Bundle By Name(cluster=w536, "G2T 2D"=w545, "G4T 2D"=w544) -> (w537:T4)
      }
      frame "Analysis: Load BG" {
        # "Template Separator\n(You can make a copy of, or modify, this frame)"
        n302 = Unbundle By Name(w600) -> ("Source Voltage"=w609:dbl, "Final Temp"=w607:i32, "Init Temp"=w604:i32, "Temp Step"=w603:i32, "Data File"=w605:path, "Trimming"=w602:i32)
        n303 = Subtract(x=w607, y=w604) -> (x-y=w610:i32)
        n304 = Divide(x=w610, y=w603) -> (x/y=w611:dbl)
        n305 = Increment(x=w611) -> (x+1=w606:dbl)
        n306 = for {
          N: w606 -> [_]
          tunnel: w609 -> [w618]
          tunnel: [w629] -> w608 mode=indexing
          tunnel: w605 -> [w628]
          tunnel: w604 -> [w627]
          tunnel: w603 -> [w626]
          tunnel: w602 -> [w625]
          i -> [w631]
          n307 = Strip Path(path=w628) -> (stripped path=w636:path, name=w635:string)
          n308 = Multiply(x=w626, y=w631) -> (x*y=w632:i32)
          n309 = Add(x=w627, y=w632) -> (x+y=w637:i32)
          n310 = String Subset(string=w635, length (rest)=18) -> (substring=w633:string)  [unwired: 1 in]
          n311 = Format Into String(w637) -> (resulting string=w639:string)  [unwired: 3 in, 1 out]
          n312 = Concatenate Strings(w633, w639, "K.dat" ("string")) -> (w638:string)
          n313 = call-poly <userlib>:"Build Path__ogtk.vi"("name or relative path"=w638, "base path"=w636) -> ("appended path"=w640:path)
          n314 = call <userlib>:"Data Read.vi"("path"=w640) -> ("Data (Dictionary)"=w623:T6[])  [unwired: 7 in, 3 out]
          n315 = call "Read Dictionary.vi"("Numeric"=0, "Dictionary In"=w623) -> ("data"=w622:dbl[])
          n316 = call "Read Dictionary.vi"("Numeric"=10, "Dictionary In"=w623) -> ("data"=w621:dbl[])
          n317 = Array Subset(array=w622, index=w625) -> (w624:dbl[])  [unwired: 1 in]
          n318 = Array Subset(array=w621, index=w625) -> (w613:dbl[])  [unwired: 1 in]
          n319 = Divide(x=w613, y=w618) -> (x/y=w617:dbl[])
          n320 = call <vilib>:"Median Filter.vi"("right rank"=-10, "left rank"=10, "X"=w617) -> ("Filtered X"=w616:dbl[])  [unwired: 7 in, 1 out]
          n321 = Bundle(w624, "Filtered X"=w616) -> (w629:cluster{dbl[], "Filtered X":dbl[]})  [unwired: 1 in]
        }
        n322 = call <vilib>:"Add State(s) to Queue__jki_lib_state_machine.vi"("State(s) in (\"\")"=w598) -> ("States Out"=w599:string)  [unwired: 14 in]
        n323 = Bundle By Name(cluster=w600, "G2T BG"=w608) -> (w601:T4)
      }
      frame "Analysis: Plot G vs t" {
        n324 = Unbundle By Name(w647) -> ("G2T 1D"=→"G2T vs t 1D":cluster{dbl[], dbl[]}[], "G4T 1D"=→"G4T vs t 1D":cluster{dbl[], dbl[]}[], "G2T 2D"=→"G2T vs t 2D":cluster{dbl[], dbl[]}[], "G4T 2D"=→"G4T vs t  2D":cluster{dbl[], dbl[]}[], "G2T BG"=→"G2T BG vs t":cluster{dbl[], dbl[]}[], "Temp"=→"Temp vs t":cluster{dbl[], dbl[]}[])
        n325 = call <vilib>:"Add State(s) to Queue__jki_lib_state_machine.vi"("State(s) in (\"\")"=w650) -> ("States Out"=w649:string)  [unwired: 14 in]
      }
      frame "Analysis: Arrhenius Plot" {
        n326 = Unbundle By Name(w691) -> ("G2T 1D"=w654:cluster{dbl[], dbl[]}[], "G4T 1D"=w653:cluster{dbl[], dbl[]}[], "G2T 2D"=w660:cluster{dbl[], dbl[]}[], "G4T 2D"=w662:cluster{dbl[], dbl[]}[], "Final Temp"=w688:i32, "Init Temp"=w686:i32, "Temp Step"=w685:i32)  [unwired: 1 out]
        n327 = Subtract(x=w688, y=w686) -> (x-y=w689:i32)
        n328 = Divide(x=w689, y=w685) -> (x/y=w690:dbl)
        n329 = Increment(x=w690) -> (x+1=w687:dbl)
        n330 = for {
          N: w687 -> [_]
          tunnel: w686 -> [w697]
          tunnel: w685 -> [w698]
          tunnel: [w695] -> w671 mode=indexing
          i -> [w699]
          n331 = Multiply(x=w698, y=w699) -> (x*y=w700:i32)
          n332 = Add(x=w697, y=w700) -> (x+y=w696:i32)
          n333 = Reciprocal(x=w696) -> (1/x=w695:dbl)
        }
        n334 = call-poly <userlib>:"Linear Fit.vi"("XY-data"=w654) -> ("slopes"=w651:dbl[])  [unwired: 4 in, 6 out]
        n335 = call-poly <userlib>:"Linear Fit.vi"("XY-data"=w653) -> ("slopes"=w652:dbl[])  [unwired: 4 in, 6 out]
        n336 = call-poly <userlib>:"Linear Fit.vi"("XY-data"=w660) -> ("slopes"=w659:dbl[])  [unwired: 4 in, 6 out]
        n337 = call-poly <userlib>:"Linear Fit.vi"("XY-data"=w662) -> ("slopes"=w661:dbl[])  [unwired: 4 in, 6 out]
        n338 = Absolute Value(x=w651) -> (abs(x)=w681:dbl[])
        n339 = Absolute Value(x=w652) -> (abs(x)=w682:dbl[])
        n340 = Absolute Value(x=w659) -> (abs(x)=w683:dbl[])
        n341 = Absolute Value(x=w661) -> (abs(x)=w684:dbl[])
        n342 = Natural Logarithm(1:w681) -> (0:w675:dbl[])
        n343 = Natural Logarithm(1:w682) -> (0:w674:dbl[])
        n344 = Natural Logarithm(1:w683) -> (0:w673:dbl[])
        n345 = Natural Logarithm(1:w684) -> (0:w672:dbl[])
        n346 = Array Subset(array=w675, length="Temps to keep (Arrhenius fit)") -> (w669:dbl[])  [unwired: 1 in]
        n347 = Array Subset(array=w674, length="Temps to keep (Arrhenius fit)") -> (w668:dbl[])  [unwired: 1 in]
        n348 = Array Subset(array=w673, length="Temps to keep (Arrhenius fit)") -> (w667:dbl[])  [unwired: 1 in]
        n349 = Array Subset(array=w672, length="Temps to keep (Arrhenius fit)") -> (w666:dbl[])  [unwired: 1 in]
        n350 = Array Subset(array=w671, length="Temps to keep (Arrhenius fit)") -> (w665:dbl[])  [unwired: 1 in]
        n351 = Bundle(w665, w669) -> (w678:cluster{dbl[], dbl[]})  [unwired: 1 in]
        n352 = Bundle(w665, w668) -> (w680:cluster{dbl[], dbl[]})  [unwired: 1 in]
        n353 = Bundle(w665, w667) -> (w679:cluster{dbl[], dbl[]})  [unwired: 1 in]
        n354 = Bundle(w665, w666) -> (w677:cluster{dbl[], dbl[]})  [unwired: 1 in]
        n355 = Build Array(w678, w680, w679, w677) -> (w658:cluster{dbl[], dbl[]}[])
        n356 = call-poly <userlib>:"Linear Fit.vi"("XY-data"=w658) -> ("Best Fits"=w657:cluster{"X-array":dbl[], "Y-array":dbl[]}[], "XY-data out"=w656:cluster{"X-array":dbl[], "Y-array":dbl[]}[], "slopes"=w655:dbl[])  [unwired: 4 in, 4 out]
        n357 = Multiply(x=w655, y=8.617333e-05) -> (x*y=→"E_a":dbl[])
        n358 = Interleave 1D Arrays(w656, w657) -> (→"Arrhenius":cluster{"X-array":dbl[], "Y-array":dbl[]}[])
        n359 = call <vilib>:"Add State(s) to Queue__jki_lib_state_machine.vi"("State(s) in (\"\")"=w694) -> ("States Out"=w693:string)  [unwired: 14 in]
      }
      frame "Analysis: Lifespan" {
        w709 = 3600
        # "Template Separator\n(You can make a copy of, or modify, this frame)"
        n360 = Unbundle By Name(w731) -> ("G2T 1D"=w748:cluster{dbl[], dbl[]}[], "G4T 1D"=w747:cluster{dbl[], dbl[]}[], "G2T 2D"=w746:cluster{dbl[], dbl[]}[], "G4T 2D"=w745:cluster{dbl[], dbl[]}[], "Final Temp"=w742:i32, "Init Temp"=w730:i32, "Temp Step"=w729:i32)  [unwired: 1 out]
        n361 = Subtract(x=w742, y=w730) -> (x-y=w743:i32)
        n362 = Divide(x=w743, y=w729) -> (x/y=w744:dbl)
        n363 = Increment(x=w744) -> (x+1=w728:dbl)
        n364 = for {
          N: w728 -> [_]
          tunnel: w730 -> [w766]
          tunnel: w729 -> [w765]
          tunnel: [w764] -> w727 mode=indexing
          i -> [w767]
          n365 = Multiply(x=w765, y=w767) -> (x*y=w768:i32)
          n366 = Add(x=w766, y=w768) -> (x+y=w764:i32)
        }
        n367 = call <userlib>:"Linear Fit (multiple).vi"("XY-data"=w748) -> ("XY-data out"=w722:cluster{"X-array":dbl[], "Y-array":dbl[]}[], "slopes"=w725:dbl[])  [unwired: 4 in, 5 out]
        n368 = call <userlib>:"Linear Fit (multiple).vi"("XY-data"=w747) -> ("XY-data out"=w721:cluster{"X-array":dbl[], "Y-array":dbl[]}[], "slopes"=w724:dbl[])  [unwired: 4 in, 5 out]
        n369 = call <userlib>:"Linear Fit (multiple).vi"("XY-data"=w746) -> ("XY-data out"=w720:cluster{"X-array":dbl[], "Y-array":dbl[]}[], "slopes"=w723:dbl[])  [unwired: 4 in, 5 out]
        n370 = call <userlib>:"Linear Fit (multiple).vi"("XY-data"=w745) -> ("XY-data out"=w719:cluster{"X-array":dbl[], "Y-array":dbl[]}[], "slopes"=w726:dbl[])  [unwired: 4 in, 5 out]
        n371 = for {
          tunnel: w722 -> [w760] mode=indexing
          tunnel: w721 -> [w761] mode=indexing
          tunnel: w720 -> [w762] mode=indexing
          tunnel: w719 -> [w763] mode=indexing
          tunnel: [w755] -> w718 mode=indexing
          tunnel: [w754] -> w717 mode=indexing
          tunnel: [w753] -> w716 mode=indexing
          tunnel: [w752] -> w715 mode=indexing
          n372 = Unbundle(w760) -> ("Y-array"=w756:dbl[])  [unwired: 1 out]
          n373 = Unbundle(w761) -> ("Y-array"=w757:dbl[])  [unwired: 1 out]
          n374 = Unbundle(w762) -> ("Y-array"=w758:dbl[])  [unwired: 1 out]
          n375 = Unbundle(w763) -> ("Y-array"=w759:dbl[])  [unwired: 1 out]
          n376 = call-poly <vilib>:"Mean.vi"("X"=w759) -> ("mean"=w752:dbl)  [unwired: 1 out]
          n377 = call-poly <vilib>:"Mean.vi"("X"=w758) -> ("mean"=w753:dbl)  [unwired: 1 out]
          n378 = call-poly <vilib>:"Mean.vi"("X"=w757) -> ("mean"=w754:dbl)  [unwired: 1 out]
          n379 = call-poly <vilib>:"Mean.vi"("X"=w756) -> ("mean"=w755:dbl)  [unwired: 1 out]
        }
        n380 = Divide(x=w718, y=w725) -> (x/y=w713:dbl[])
        n381 = Divide(x=w717, y=w724) -> (x/y=w712:dbl[])
        n382 = Divide(x=w716, y=w723) -> (x/y=w711:dbl[])
        n383 = Divide(x=w715, y=w726) -> (x/y=w710:dbl[])
        n384 = Divide(x=w713, y=w709) -> (x/y=w705:dbl[])
        n385 = Divide(x=w712, y=w709) -> (x/y=w706:dbl[])
        n386 = Divide(x=w711, y=w709) -> (x/y=w707:dbl[])
        n387 = Divide(x=w710, y=w709) -> (x/y=w708:dbl[])
        n388 = Array Subset(array=w705, length="Temps to keep (Lifespan)") -> (w736:dbl[])  [unwired: 1 in]
        n389 = Array Subset(array=w706, length="Temps to keep (Lifespan)") -> (w735:dbl[])  [unwired: 1 in]
        n390 = Array Subset(array=w707, length="Temps to keep (Lifespan)") -> (w734:dbl[])  [unwired: 1 in]
        n391 = Array Subset(array=w708, length="Temps to keep (Lifespan)") -> (w733:dbl[])  [unwired: 1 in]
        n392 = Array Subset(array=w727, length="Temps to keep (Lifespan)") -> (w732:i32[])  [unwired: 1 in]
        n393 = Absolute Value(x=w736) -> (abs(x)=w701:dbl[])
        n394 = Absolute Value(x=w735) -> (abs(x)=w702:dbl[])
        n395 = Absolute Value(x=w734) -> (abs(x)=w703:dbl[])
        n396 = Absolute Value(x=w733) -> (abs(x)=w704:dbl[])
        n397 = Bundle(w732, w701) -> (w739:cluster{i32[], dbl[]})  [unwired: 1 in]
        n398 = Bundle(w732, w702) -> (w741:cluster{i32[], dbl[]})  [unwired: 1 in]
        n399 = Bundle(w732, w703) -> (w740:cluster{i32[], dbl[]})  [unwired: 1 in]
        n400 = Bundle(w732, w704) -> (w738:cluster{i32[], dbl[]})  [unwired: 1 in]
        n401 = Build Array(w739, w741, w740, w738) -> (→"Lifespan vs Temp (hrs)":cluster{i32[], dbl[]}[])
        n402 = call <vilib>:"Add State(s) to Queue__jki_lib_state_machine.vi"("State(s) in (\"\")"=w751) -> ("States Out"=w750:string)  [unwired: 14 in]
      }
    }
  }
  "error out" <- w1
